vi "LIA Fgen Dual Channel.vi"() -> ()   [LabVIEW 2017]
doc: "This example shows how to use the Arbitrary Waveform mode to generate on two channels."
uses:
  <instrlib>/niFgen/niFgen.llb/niFgen Output Mode.ctl
  <instrlib>/niFgen/niFgen.llb/niFgen Waveform Type.ctl
panel:
  in  "Frequency":dbl=100000.0 format="%_6p"
  in  "Amplitude":dbl=1.0 format="%_8g"
  in  "Stop":bool
  in  "FGEN Resource Name":refnum<k15>="Dev4"
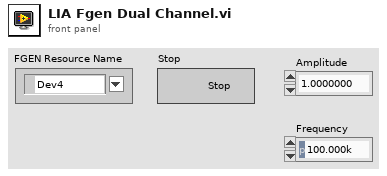
[diagram p1: front panel]
types:
  T1 = typedef "niFgen Waveform Type.ctl" = i32
  T2 = typedef "niFgen Output Mode.ctl" = u32
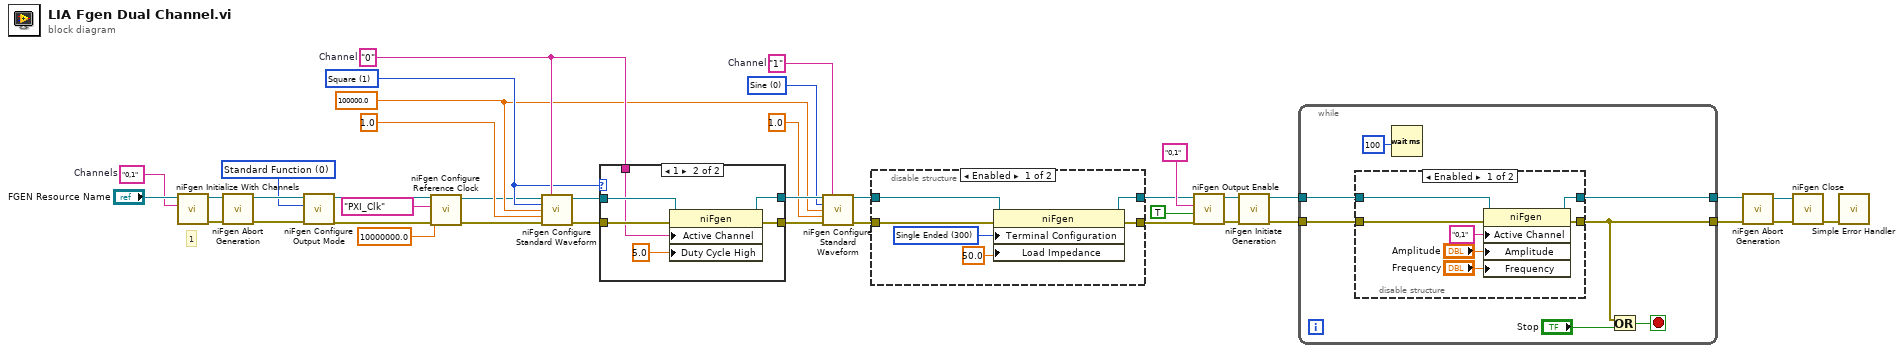
[diagram p0: block diagram]
diagram:
  w17 = "1"  # Channel
  w19 = T1 0 items=["Sine", "Square", "Triangle", "Ramp Up", "Ramp Down", "DC", "Noise", "User"] ("Waveform")
  w6 = 100000.0 ("Frequency")
  w7 = T1 1 items=["Sine", "Square", "Triangle", "Ramp Up", "Ramp Down", "DC", "Noise", "User"] ("Waveform")
  w24 = "0"  # Channel
  w30 = T2 0 items=["Standard Function", "Frequency List", "Arbitrary Waveform", "Arbitrary Sequence", "Script"] ("Output Mode")
  w35 = "0,1"  # Channels
  # "1"
  n1 = call <instrlib>:"niFgen Initialize With Channels.vi"("Channel Name"=w35, "Resource Name"="FGEN Resource Name") -> ("error out"=w34:errorcluster, "Instrument Handle Out"=w33:refnum<k15>)  [unwired: 8 in]
  n2 = call <instrlib>:"niFgen Abort Generation.vi"("error in (no error)"=w34, "Instrument Handle"=w33) -> ("error out"=w32:errorcluster, "Instrument Handle Out"=w31:refnum<k15>)  [unwired: 8 in]
  n3 = call <instrlib>:"niFgen Configure Output Mode.vi"("error in (no error)"=w32, "Output Mode (default: 0=Standard Function)"=w30, "Instrument Handle"=w31) -> ("error out"=w26:errorcluster, "Instrument Handle Out"=w4:refnum<k15>)  [unwired: 6 in]
  n4 = call <instrlib>:"niFgen Configure Reference Clock.vi"("error in (no error)"=w26, "Reference Clock Frequency"=10000000.0, "Source"="PXI_Clk", "Instrument Handle"=w4) -> ("error out"=w5:errorcluster, "Instrument Handle Out"=w3:refnum<k15>)  [unwired: 6 in]
  n5 = call <instrlib>:"niFgen Configure Standard Waveform.vi"("Instrument Handle"=w3, "Channel Name"=w24, "Waveform"=w7, "Frequency"=w6, "Amplitude"=1.0, "error in (no error)"=w5) -> ("Instrument Handle Out"=w28:refnum<k15>, "error out"=w27:errorcluster)  [unwired: 8 in]
  n6 = case shown="1" w7 {
    tunnel: w28 -> [w41 w47]
    tunnel: w27 -> [w40 w46]
    tunnel: w24 -> [_ w45]
    tunnel: [w41 w43] -> w20
    tunnel: [w40 w42] -> w16
    frame Default {
    }
    frame 1 {
      n7 = property class="niFgen"(reference=w47, error in=w46, "Active Channel"=w45, "Duty Cycle High"=5.0 ("Standard Function:Duty Cycle High")) -> (reference out=w43:refnum<k15>, error out=w42:errorcluster)
    }
  }
  n8 = call <instrlib>:"niFgen Configure Standard Waveform.vi"("Instrument Handle"=w20, "Channel Name"=w17, "Waveform"=w19, "Frequency"=w6, "Amplitude"=1.0, "error in (no error)"=w16) -> ("Instrument Handle Out"=w9:refnum<k15>, "error out"=w15:errorcluster)  [unwired: 8 in]
  n9 = disable-structure shown="Enabled" {
    disable-tunnel: w15 -> [w53 w54]
    disable-tunnel: [w52 w54] -> w10
    disable-tunnel: w9 -> [w51 w55]
    disable-tunnel: [w50 w55] -> w8
    frame Enabled {
      w49 = 300 items=["Single Ended"=300, "Differential"=301] ("Output:Terminal Configuration")
      n10 = property class="niFgen"(reference=w51, error in=w53, "Terminal Configuration"=w49, "Load Impedance"=50.0 ("Output:Load Impedance")) -> (reference out=w50:refnum<k15>, error out=w52:errorcluster)
    }
    frame Disabled {
    }
  }
  n11 = call <instrlib>:"niFgen Output Enable.vi"("error in (no error)"=w10, "Output Enable (default: True)"=TRUE ("output enable"), "Channel Name"="0,1", "Instrument Handle"=w8) -> ("error out"=w21:errorcluster, "Instrument Handle Out"=w22:refnum<k15>)  [unwired: 6 in]
  n12 = call <instrlib>:"niFgen Initiate Generation.vi"("error in (no error)"=w21, "Instrument Handle"=w22) -> ("error out"=w13:errorcluster, "Instrument Handle Out"=w11:refnum<k15>)  [unwired: 8 in]
  n13 = while {
    tunnel: [w58] -> w14
    tunnel: w13 -> [w59]
    tunnel: [w56] -> w12
    tunnel: w11 -> [w57]
    stop <- w60 stop-if-true
    n14 = disable-structure shown="Enabled" {
      disable-tunnel: w59 -> [w69 w70]
      disable-tunnel: [w68 w70] -> w58
      disable-tunnel: w57 -> [w67 w71]
      disable-tunnel: [w66 w71] -> w56
      frame Enabled {
        n15 = property class="niFgen"(reference=w67, error in=w69, "Active Channel"="0,1", "Amplitude"="Amplitude", "Frequency"="Frequency") -> (reference out=w66:refnum<k15>, error out=w68:errorcluster)
      }
      frame Disabled {
      }
    }
    n16 = Wait (ms)(milliseconds to wait=u32 100 ("millisecond multiple")) -> ()  [unwired: 1 out]
    n17 = Or(x=w58, y="Stop") -> (x .or. y?=w60:bool)
  }
  n18 = call <instrlib>:"niFgen Abort Generation.vi"("error in (no error)"=w14, "Instrument Handle"=w12) -> ("error out"=w39:errorcluster, "Instrument Handle Out"=w38:refnum<k15>)  [unwired: 8 in]
  n19 = call <instrlib>:"niFgen Close.vi"("error in (no error)"=w39, "Instrument Handle"=w38) -> ("error out"=w37:errorcluster)  [unwired: 9 in]
  n20 = call <vilib>:"Simple Error Handler.vi"("error in (no error)"=w37) -> ()  [unwired: 4 in, 5 out]
